vi "Build Frame Script Core.vi"(8 "error in (no error)":errorcluster, 10 "Config Strings":string[](array[string]), 11 "BML_LS Pattern Creator in":refnum<class "BML_LS Pattern Creator.lvclass">) -> (0 "error out":errorcluster, 2 "Pattern Script":string, 3 "BML_LS Pattern Creator out":refnum<class "BML_LS Pattern Creator.lvclass">)   [LabVIEW 2018, in "BML_LS Pattern Creator.lvlib" / "BML_LS Pattern Creator.lvclass"]
uses:
  BML_LS Pattern Creator.lvclass
  Protocols/BML Pattern Creater.lvlibp/Plugins/SouceCode/BML Pattern Creater/BML Pattern Creater.lvclass
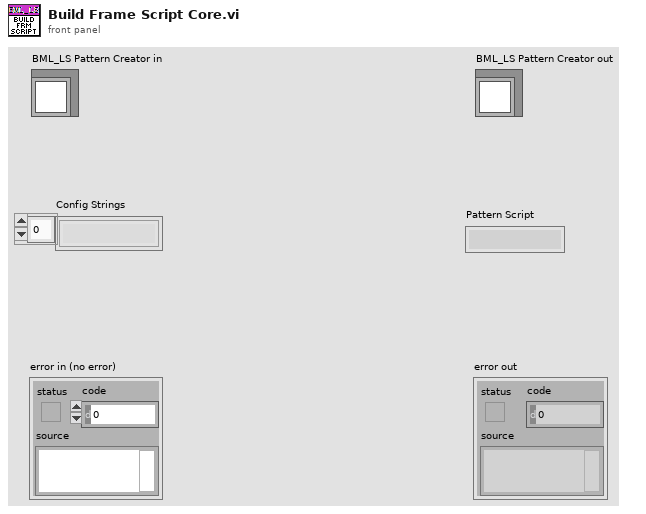
[diagram p1: front panel]
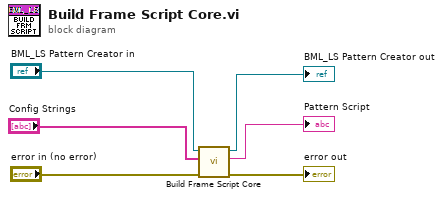
[diagram p0: block diagram]
diagram:
  n1 = call-parent "Build Frame Script Core.vi"("error in (no error)"="error in (no error)", "Config Strings"="Config Strings", "BML Pattern Creater in"="BML_LS Pattern Creator in") -> ("error out"=→"error out":errorcluster, "Pattern Script"=→"Pattern Script":string, "BML Pattern Creater out"=→"BML_LS Pattern Creator out":refnum<class "BML_LS Pattern Creator.lvclass">)  [unwired: 6 in]
